vi "Train Magnet.vi"(8 "error in (no error)":errorcluster, 11 "Power Supply in":refnum<class "Power Supply.lvclass">) -> (0 "error out":errorcluster, 2 "This VI":refnum<vi>, 3 "Power Supply out":refnum<class "Power Supply.lvclass">)   [LabVIEW 2015, in "Power Supply.lvclass"]
uses:
  Power Supply.lvclass
  Power Supply.lvclass/Power Supply.ctl
  Global/Relative Sound Files.vi
panel:
  out "Done":bool
  out "Training":bool
  out "original rate":dbl[unit] caption="Original Rate"
  out "going to field? (false when at field)":bool
  out "going up?":bool
  out "currently going to field":dbl[unit]
  out "current field":dbl[unit]
  out "active":bool
  out "rate":dbl[unit] caption="Current Rate"
  in  "interrupt":bool
  out "Original Field":dbl[unit]
  in  "endprogram":bool
  in  "go":bool
  in  "upanddown":bool=TRUE
  in  "Train to Field":dbl[unit]=7.0
  # "To what field would you like to train the magnet?"
  # "Training means going up to the desired field at the \"train speed\"\nand then coming back down to the starting field, again, at the \"train speed.\" Going to 7 T takes about 42 min, one way."
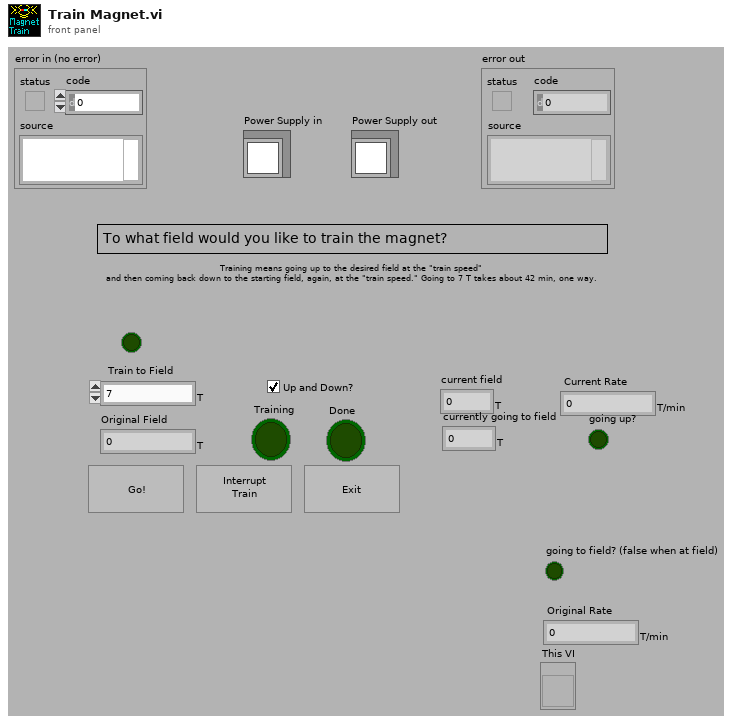
[diagram p1: front panel]
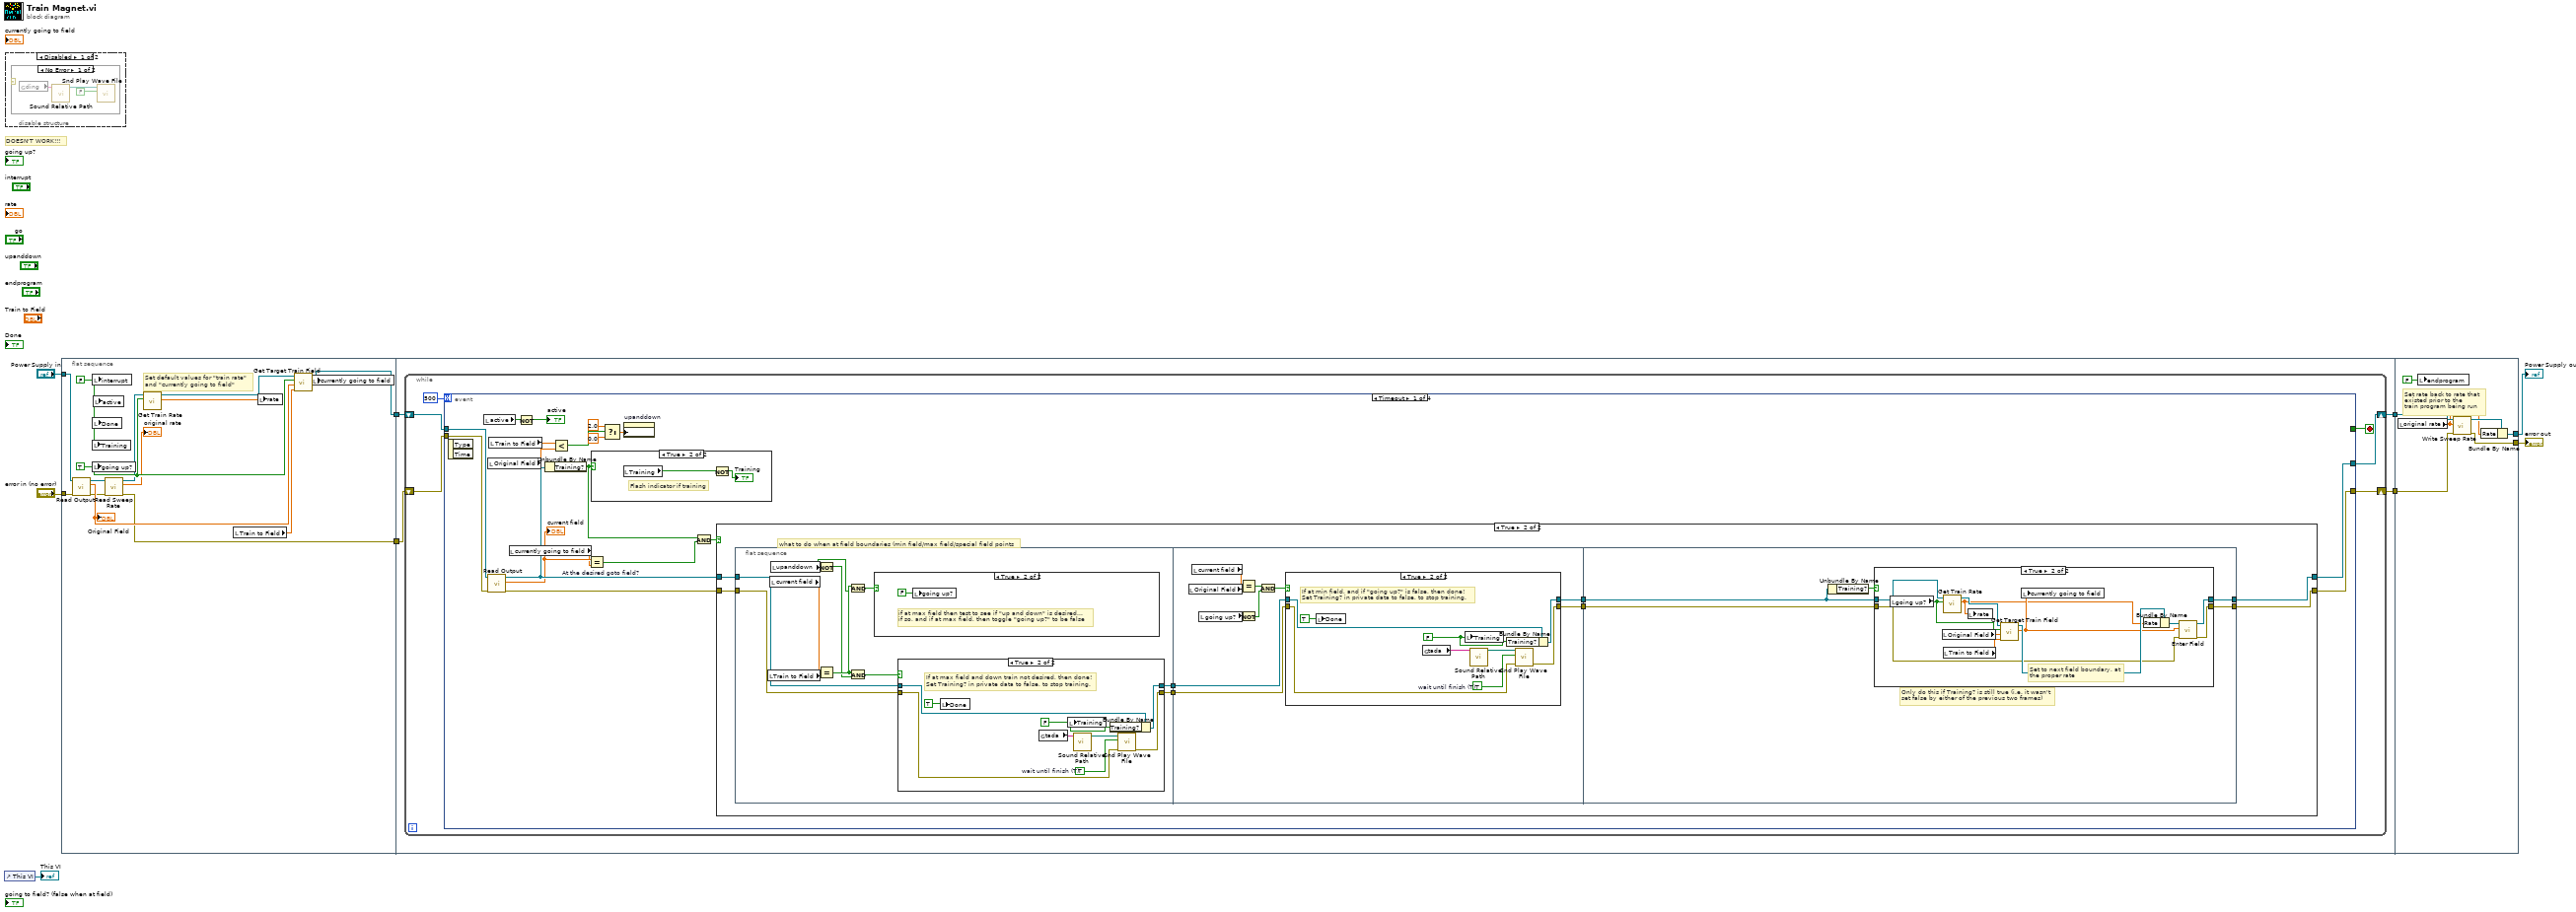
[diagram p0: block diagram]
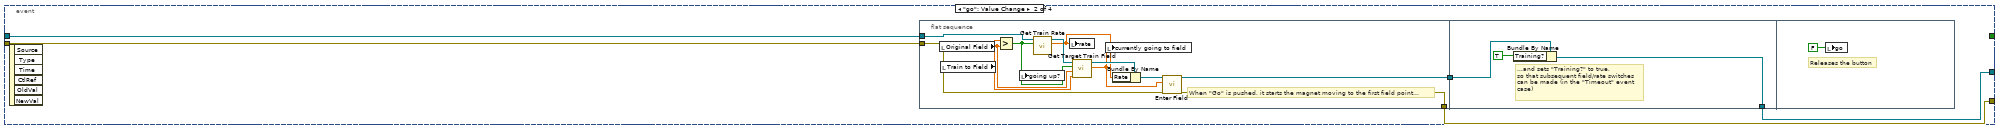
[diagram p10: hidden frame]
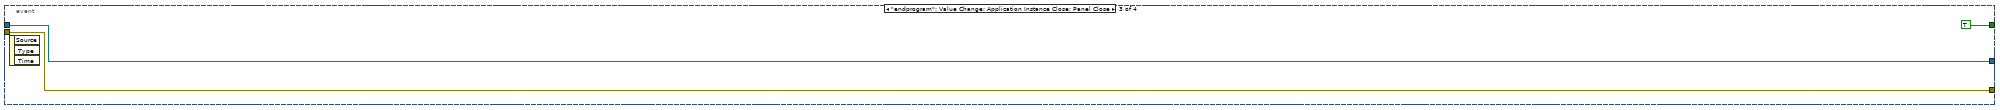
[diagram p11: hidden frame]
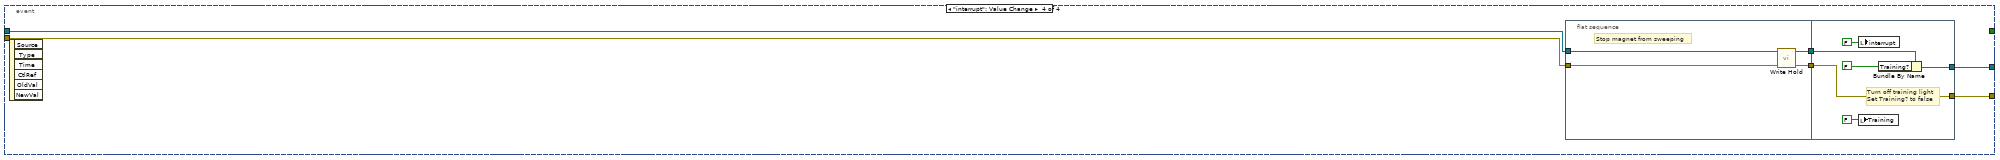
[diagram p12: hidden frame]
diagram:
  # "DOESN'T WORK!!!"
  n1 = control-ref of="This VI"() -> (→"This VI":refnum<vi>)
  n2 = disable-structure shown="Disabled" {
    frame Disabled {
      n3 = case shown="No Error" {
        selector: _ -> [_ _]
        frame No Error {
          n4 = global read "Relative Sound Files.vi" "ding"() -> (w11:string)
          n5 = call "Sound Relative Path.vi"("Sound"=w11) -> ("Relative Path"=w10:path)  [unwired: 10 in]
          n6 = call <vilib>:"Snd Play Wave File.vi"("wait until finish (T)"=FALSE, "wave file path"=w10) -> ()  [unwired: 1 in, 9 out]
        }
        frame Error {
        }
      }
    }
    frame Enabled {
    }
  }
  n7 = flat-sequence {
    tunnel: "Power Supply in" -> [w27]
    tunnel: "error in (no error)" -> [w26]
    tunnel: [w20] -> w6
    tunnel: [w16] -> w5
    tunnel: [w31] -> w4
    tunnel: [w30] -> w3
    tunnel: w6 -> [w29]
    tunnel: w5 -> [w28]
    tunnel: w4 -> [w176]
    tunnel: [w177] -> w9
    tunnel: w3 -> [w173]
    tunnel: [w172] -> w2
    frame #0 {
      w23 = TRUE ("going up?")
      w13 = FALSE
      # "Set default values for \"train rate\"\nand \"currently going to field\""
      n8 = call-dynamic "Read Output.vi"("error in (no error)"=w26, "Power Supply in"=w27) -> ("error out"=w17:errorcluster, "Field"=w22:dbl[unit], "Power Supply out"=w19:refnum<class "Power Supply.lvclass">)  [unwired: 5 in, 2 out]
      "Original Field" <- w22
      n9 = local write "Training"(w13) -> ()
      n10 = local write "going up?"(w23) -> ()
      n11 = local write "interrupt"(w13) -> ()
      n12 = local write "Done"(w13) -> ()
      n13 = local write "active"(w13) -> ()
      n14 = call-dynamic "Read Sweep Rate.vi"("error in (no error)"=w17, "Power Supply in"=w19) -> ("error out"=w16:errorcluster, "Field sweep rate"=→"original rate":dbl[unit], "Power Supply out"=w18:refnum<class "Power Supply.lvclass">)  [unwired: 7 in]
      n15 = call "Get Train Rate.vi"("going up?"=w23, "Power Supply in"=w18) -> ("Rate Out"=w24:dbl[unit], "Power Supply Out"=w25:refnum<class "Power Supply.lvclass">)  [unwired: 8 in]
      n16 = local read "Train to Field"() -> (w21:dbl[unit])
      n17 = local write "rate"(w24) -> ()
      n18 = call "Get Target Train Field.vi"("Train to Field"=w21, "Original Field"=w22, "going up?"=w23, "Power Supply in"=w25) -> ("Target Field"=w14:dbl[unit], "Power Supply Out"=w20:refnum<class "Power Supply.lvclass">)  [unwired: 6 in]
      n19 = local write "currently going to field"(w14) -> ()
    }
    frame #1 {
      n20 = while {
        shift-right: [w34] -> w31
        shift-left: w29 -> [w35]
        shift-right: [w33] -> w30
        shift-left: w28 -> [w32]
        stop <- w37 stop-if-true
        n21 = event shown="[0] Timeout" {
          selector: _ -> [_ _ _ _]
          dyn-events: _ -> [_ _ _ _]
          timeout: 500 -> [_ _ _ _]
          tunnel: [_ _ TRUE ("endprogram") _] -> w37
          tunnel: w35 -> [w54 w135 w155 w161]
          tunnel: [w52 w136 w155 w156] -> w34
          tunnel: [w50 w132 w154 w159] -> w33
          tunnel: w32 -> [w53 w133 w154 w160]
          event Timeout {
            n22 = event-data() -> ()  [unwired: 3 out]
            n23 = local read "active"() -> (w56:bool)
            n24 = local read "Original Field"() -> (w40:dbl[unit])
            n25 = call-dynamic "Read Output.vi"("error in (no error)"=w53, "Power Supply in"=w54) -> ("error out"=w51:errorcluster, "Field"=w47:dbl[unit], "Power Supply out"=w49:refnum<class "Power Supply.lvclass">)  [unwired: 5 in, 2 out]
            "current field" <- w47
            n26 = local read "Train to Field"() -> (w41:dbl[unit])
            n27 = local read "currently going to field"() -> (w46:dbl[unit])
            n28 = Not(x=w56) -> (.not. x?=→"active":bool)
            n29 = Unbundle By Name(w49) -> ("Training?"=w44:bool)
            n30 = Less?(x=w41, y=w40) -> (x < y?=w39:bool)
            n31 = Equal? "At the desired goto field?"(x=w47, y=w46) -> (x = y?=w45:bool)
            n32 = case shown="True" w44 {
              frame False {
              }
              frame True {
                # "Flash indicator if training"
                n33 = local read "Training"() -> (w57:bool)
                n34 = Not(x=w57) -> (.not. x?=→"Training":bool)
              }
            }
            n35 = Select(t=2.0 ("f"), s=w39, f=0.0) -> (s? t:f=w38:dbl)
            n36 = property on="upanddown" class="Bool (strict)"("DisabledEnum"=w38) -> ()  [unwired: 2 in, 2 out]
            n37 = And(x=w44, y=w45) -> (x .and. y?=w48:bool)
            n38 = case shown="True" w48 {
              tunnel: w51 -> [w59 w61]
              tunnel: [w59 w68] -> w50
              tunnel: w49 -> [w60 w67]
              tunnel: [w60 w66] -> w52
              frame False {
              }
              frame True {
                # "what to do when at field boundaries (min field/max field/special field points"
                n39 = flat-sequence {
                  tunnel: [w71] -> w65
                  tunnel: w67 -> [w72]
                  tunnel: [w69] -> w62
                  tunnel: w61 -> [w70]
                  tunnel: w65 -> [w95]
                  tunnel: [w94] -> w64
                  tunnel: [w92] -> w63
                  tunnel: w62 -> [w93]
                  tunnel: [w117] -> w66
                  tunnel: [w116] -> w68
                  tunnel: w64 -> [w115]
                  tunnel: w63 -> [w113]
                  frame #0 {
                    n40 = local read "Train to Field"() -> (w78:dbl[unit])
                    n41 = local read "current field"() -> (w79:dbl[unit])
                    n42 = local read "upanddown"() -> (w74:bool)
                    n43 = Not(x=w74) -> (.not. x?=w75:bool)
                    n44 = Equal?(x=w79, y=w78) -> (x = y?=w76:bool)
                    n45 = And(x=w76, y=w74) -> (x .and. y?=w77:bool)
                    n46 = And(x=w76, y=w75) -> (x .and. y?=w73:bool)
                    n47 = case shown="True" w77 {
                      frame False {
                      }
                      frame True {
                        # "if at max field then test to see if \"up and down\" is desired... \nif so, and if at max field, then toggle \"going up?\" to be false"
                        n48 = local write "going up?"(FALSE ("going up?")) -> ()
                      }
                    }
                    n49 = case shown="True" w73 {
                      tunnel: w72 -> [w81 w90]
                      tunnel: [w81 w89] -> w71
                      tunnel: w70 -> [w80 w83]
                      tunnel: [w80 w82] -> w69
                      frame False {
                      }
                      frame True {
                        w86 = TRUE  # wait until finish (T)
                        w87 = FALSE ("Training?")
                        # "If at max field and down train not desired, then done!\nSet Training? in private data to false, to stop training."
                        n50 = local write "Done"(TRUE ("Done")) -> ()
                        n51 = global read "Relative Sound Files.vi" "tada"() -> (w84:string)
                        n52 = local write "Training"(w87) -> ()
                        n53 = call "Sound Relative Path.vi"("Sound"=w84) -> ("Relative Path"=w85:path)  [unwired: 10 in]
                        n54 = Bundle By Name(cluster=w90, "Training?"=w87) -> (w89:refnum<class "Power Supply.lvclass">)
                        n55 = call <vilib>:"Snd Play Wave File.vi"("error in (no error)"=w83, "wait until finish (T)"=w86, "wave file path"=w85) -> ("error out"=w82:errorcluster)  [unwired: 8 out]
                      }
                    }
                  }
                  frame #1 {
                    n56 = local read "Original Field"() -> (w98:dbl[unit])
                    n57 = local read "current field"() -> (w97:dbl[unit])
                    n58 = local read "going up?"() -> (w101:bool)
                    n59 = Equal?(x=w97, y=w98) -> (x = y?=w99:bool)
                    n60 = Not(x=w101) -> (.not. x?=w100:bool)
                    n61 = And(x=w99, y=w100) -> (x .and. y?=w96:bool)
                    n62 = case shown="True" w96 {
                      tunnel: w95 -> [w103 w112]
                      tunnel: [w103 w111] -> w94
                      tunnel: w93 -> [w102 w105]
                      tunnel: [w102 w104] -> w92
                      frame False {
                      }
                      frame True {
                        w108 = TRUE  # wait until finish (T)
                        w109 = FALSE ("Training?")
                        # "If at min field, and if \"going up?\" is false, then done!\nSet Training? in private data to false, to stop training."
                        n63 = local write "Done"(TRUE ("Done")) -> ()
                        n64 = global read "Relative Sound Files.vi" "tada"() -> (w106:string)
                        n65 = local write "Training"(w109) -> ()
                        n66 = call "Sound Relative Path.vi"("Sound"=w106) -> ("Relative Path"=w107:path)  [unwired: 10 in]
                        n67 = Bundle By Name(cluster=w112, "Training?"=w109) -> (w111:refnum<class "Power Supply.lvclass">)
                        n68 = call <vilib>:"Snd Play Wave File.vi"("error in (no error)"=w105, "wait until finish (T)"=w108, "wave file path"=w107) -> ("error out"=w104:errorcluster)  [unwired: 8 out]
                      }
                    }
                  }
                  frame #2 {
                    # "Only do this if Training? is still true (i.e. it wasn't \nset false by either of the previous two frames)"
                    n69 = Unbundle By Name(w115) -> ("Training?"=w114:bool)
                    n70 = case shown="True" w114 {
                      tunnel: w113 -> [w118 w125]
                      tunnel: [w119 w124] -> w117
                      tunnel: [w118 w123] -> w116
                      tunnel: w115 -> [w119 w122]
                      frame False {
                      }
                      frame True {
                        # "Set to next field boundary, at\nthe proper rate"
                        n71 = local read "going up?"() -> (w129:bool)
                        n72 = local read "Original Field"() -> (w127:dbl[unit])
                        n73 = call "Get Train Rate.vi"("going up?"=w129, "Power Supply in"=w122) -> ("Rate Out"=w120:dbl[unit], "Power Supply Out"=w126:refnum<class "Power Supply.lvclass">)  [unwired: 8 in]
                        n74 = local read "Train to Field"() -> (w128:dbl[unit])
                        n75 = local write "rate"(w120) -> ()
                        n76 = call "Get Target Train Field.vi"("Train to Field"=w128, "Original Field"=w127, "going up?"=w129, "Power Supply in"=w126) -> ("Target Field"=w121:dbl[unit], "Power Supply Out"=w130:refnum<class "Power Supply.lvclass">)  [unwired: 6 in]
                        n77 = local write "currently going to field"(w121) -> ()
                        n78 = Bundle By Name(cluster=w130, "Rate"=w120) -> (w131:refnum<class "Power Supply.lvclass">)
                        n79 = call-dynamic "Enter Field.vi"("error in (no error)"=w125, "Target field"=w121, "Power Supply in"=w131) -> ("error out"=w123:errorcluster, "Power Supply out"=w124:refnum<class "Power Supply.lvclass">)  [unwired: 7 in]
                      }
                    }
                  }
                }
              }
            }
          }
          event "go": Value Change {
            n80 = event-data() -> ()  [unwired: 7 out]
            n81 = flat-sequence {
              tunnel: [w142] -> w134
              tunnel: [w140] -> w132
              tunnel: w135 -> [w143]
              tunnel: w133 -> [w141]
              tunnel: [w150] -> w136
              tunnel: w134 -> [w149]
              frame #0 {
                # "When \"Go\" is pushed, it starts the magnet moving to the first field point..."
                n82 = local read "Original Field"() -> (w138:dbl[unit])
                n83 = local read "Train to Field"() -> (w139:dbl[unit])
                n84 = Greater?(x=w139, y=w138) -> (0:w137:bool)
                n85 = local write "going up?"(w137) -> ()
                n86 = call "Get Train Rate.vi"("going up?"=w137, "Power Supply in"=w143) -> ("Rate Out"=w144:dbl[unit], "Power Supply Out"=w146:refnum<class "Power Supply.lvclass">)  [unwired: 8 in]
                n87 = local write "rate"(w144) -> ()
                n88 = call "Get Target Train Field.vi"("Train to Field"=w139, "Original Field"=w138, "going up?"=w137, "Power Supply in"=w146) -> ("Target Field"=w145:dbl[unit], "Power Supply Out"=w147:refnum<class "Power Supply.lvclass">)  [unwired: 6 in]
                n89 = local write "currently going to field"(w145) -> ()
                n90 = Bundle By Name(cluster=w147, "Rate"=w144) -> (w148:refnum<class "Power Supply.lvclass">)
                n91 = call-dynamic "Enter Field.vi"("error in (no error)"=w141, "Target field"=w145, "Power Supply in"=w148) -> ("error out"=w140:errorcluster, "Power Supply out"=w142:refnum<class "Power Supply.lvclass">)  [unwired: 7 in]
              }
              frame #1 {
                # "...and sets \"Training?\" to true,\nso that subsequent field/rate switches\ncan be made (in the \"Timeout\" event \ncase)"
                n92 = Bundle By Name(cluster=w149, "Training?"=TRUE) -> (w150:refnum<class "Power Supply.lvclass">)
              }
              frame #2 {
                # "Releases the button"
                n93 = local write "go"(FALSE ("go")) -> ()
              }
            }
          }
          event "endprogram": Value Change; Application Instance Close; Panel Close {
            n94 = event-data() -> ()  [unwired: 4 out]
          }
          event "interrupt": Value Change {
            n95 = event-data() -> ()  [unwired: 7 out]
            n96 = flat-sequence {
              tunnel: w161 -> [w165]
              tunnel: w160 -> [w164]
              tunnel: [w163] -> w158
              tunnel: [w162] -> w157
              tunnel: [w171] -> w159
              tunnel: w158 -> [w171]
              tunnel: [w168] -> w156
              tunnel: w157 -> [w167]
              frame #0 {
                # "Stop magnet from sweeping"
                n97 = call-dynamic "Write Hold.vi"("error in (no error)"=w164, "Power Supply in"=w165) -> ("error out"=w163:errorcluster, "Power Supply out"=w162:refnum<class "Power Supply.lvclass">)  [unwired: 8 in]
              }
              frame #1 {
                # "Turn off training light\nSet Training? to false"
                n98 = local write "Training"(FALSE ("Training")) -> ()
                n99 = local write "interrupt"(FALSE) -> ()
                n100 = Bundle By Name(cluster=w167, "Training?"=FALSE) -> (w168:refnum<class "Power Supply.lvclass">)
              }
            }
          }
        }
      }
    }
    frame #2 {
      # "Set rate back to rate that\nexisted prior to the \ntrain program being run"
      n101 = local read "original rate"() -> (w174:dbl[unit])
      n102 = local write "endprogram"(FALSE) -> ()
      n103 = call-dynamic "Write Sweep Rate.vi"("error in (no error)"=w173, "rate"=w174, "Power Supply in"=w176) -> ("error out"=w172:errorcluster, "Power Supply out"=w175:refnum<class "Power Supply.lvclass">)  [unwired: 7 in]
      n104 = Bundle By Name(cluster=w175, "Rate"=w174) -> (w177:refnum<class "Power Supply.lvclass">)
    }
  }
  "Power Supply out" <- w9
  "error out" <- w2
